vi "Z900_navX_SERIAL_ValidatePacketTermination.vi"(2 "Expected Packet Length":i32, 3 "Buffer":string) -> (0 "Packet Termination Offset":i32, 1 "Packet Valid":bool)   [LabVIEW 2015, in "navX Library v2.lvlib"]
uses:
  navX Library v2.lvlib
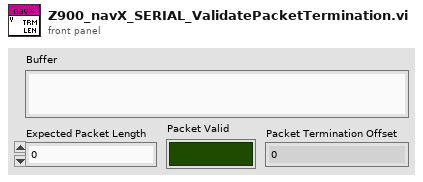
[diagram p1: front panel]
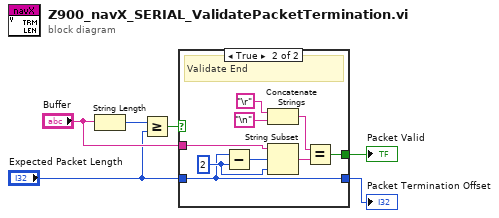
[diagram p0: block diagram]
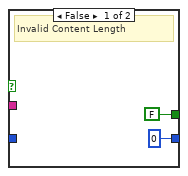
[diagram p2: hidden frame]
diagram:
  n1 = String Length(string="Buffer") -> (length=w6:i32)
  n2 = Greater Or Equal?(x=w6, y="Expected Packet Length") -> (x >= y?=w5:bool)
  n3 = case shown="True" w5 {
    tunnel: "Expected Packet Length" -> [_ w9]
    tunnel: "Buffer" -> [_ w14]
    tunnel: [FALSE w11] -> w2
    tunnel: [0 ("Expected Packet Length") w9] -> w1
    frame False {
      # "Invalid Content Length"
    }
    frame True {
      w13 = 2 ("length (rest)")
      # "Validate End"
      n4 = Subtract(x=w9, y=w13) -> (x-y=w10:i32)
      n5 = Concatenate Strings("\r", "\n") -> (w15:string)
      n6 = String Subset(string=w14, offset (0)=w10, length (rest)=w13) -> (substring=w12:string)
      n7 = Equal?(x=w15, y=w12) -> (x = y?=w11:bool)
    }
  }
  "Packet Valid" <- w2
  "Packet Termination Offset" <- w1
